vi "Init Hardware.vi"(8 "error in (no error)":errorcluster, 11 "rotator driver in":refnum<class "rotator driver.lvclass">) -> (0 "error out":errorcluster, 3 "rotator driver out":refnum<class "rotator driver.lvclass">)   [LabVIEW 2020, in "rotator driver.lvclass"]
uses:
  rotator driver.lvclass
  opt/github/NHMFL_Core/Libraries/Instruments/VISA Instrument/VISA Instrument.lvclass
  stepper driver action.ctl
  NHMFL_Core/Libraries/Instruments/VISA Instrument/VISA Instrument.lvclass/VISA Instrument.ctl
  NHMFL_Core/Libraries/Instruments/VISA Instrument/Read VISA resource.vi
  stepper driver -- BLM.vi
  rotator driver.lvclass/rotator driver.ctl
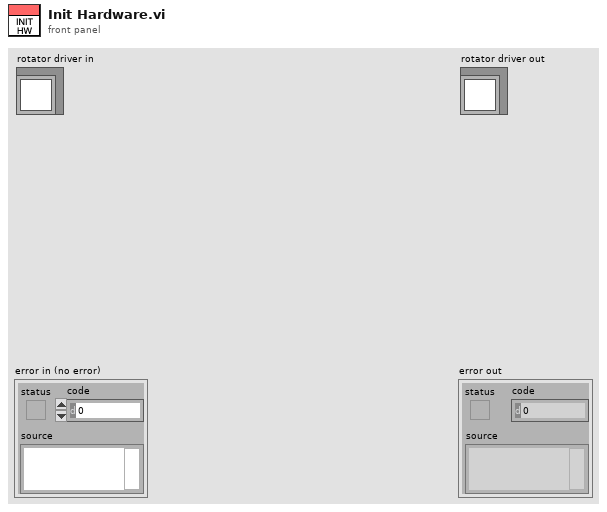
[diagram p1: front panel]
types:
  T1 = typedef "stepper driver action.ctl" = enum16{"go", "void", "stop", "check", "init", "sync", "set", "set speed", "--check status", "--check value", "--handshake"}
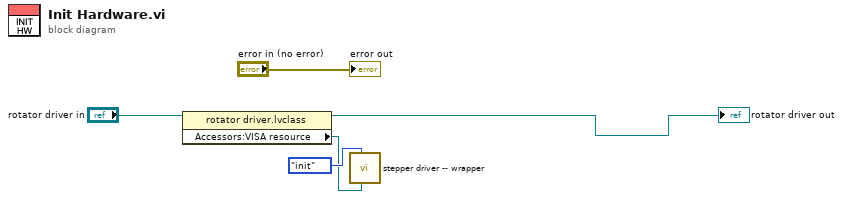
[diagram p0: block diagram]
diagram:
  n1 = property class="rotator driver.lvclass"(reference="rotator driver in") -> (reference out=→"rotator driver out":refnum<class "rotator driver.lvclass">, "Accessors:VISA resource"=w2:refnum<visa-resource-name>)  [unwired: 1 in, 1 out]
  n2 = call "stepper driver -- wrapper.vi"("Instrument Address"=w2, "stepper driver action"=stepper_driver_action."init") -> ()  [unwired: 7 in, 3 out]
  "error out" <- "error in (no error)"
